vi "Utility Default Instrument Setup.vi"(0 "VISA resource name":refnum<visa-resource-name>, 11 "error in (no error)":errorcluster) -> (4 "VISA resource name out":refnum<visa-resource-name>, 15 "error out":errorcluster)   [LabVIEW 2016, in "Fluke 5XXX Series Multicalibrators.lvlib"]
doc: "This Utility VI sends a default command string to the instrument whenever a new VISA session is opened, or the instrument is reset. This VI is intended to be used as a subVI for the FL5XMCAL Initialize and FL5XMCAL Reset VI's. Altering this VI could cause these two VI's to operate incorrectly."
uses:
  Fluke 5XXX Series Multicalibrators.lvlib
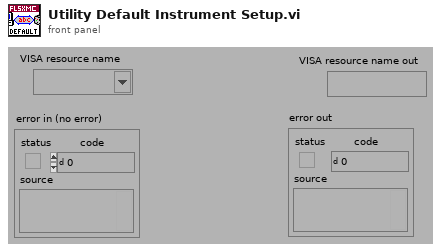
[diagram p1: front panel]
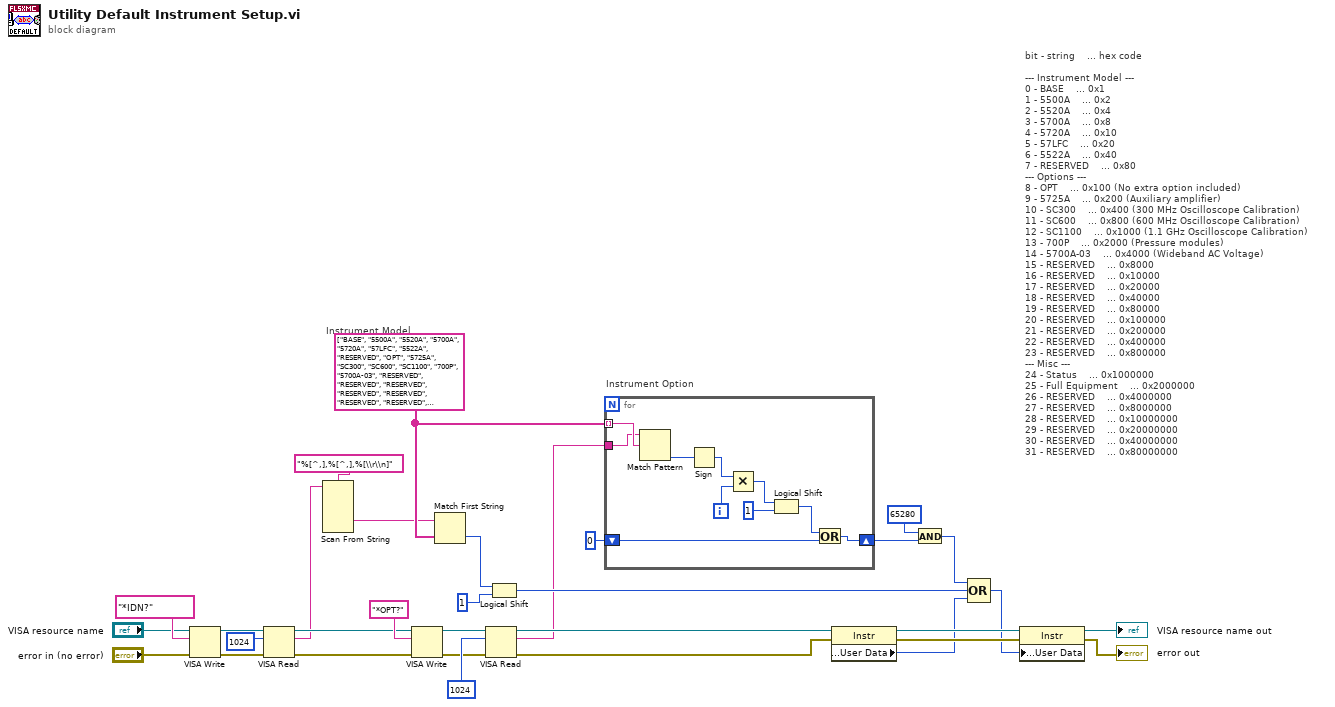
[diagram p0: block diagram]
diagram:
  w16 = string[] ["BASE", "5500A", "5520A", "5700A", "5720A", "57LFC", "5522A", "RESERVED", "OPT", "5725A", "SC300", "SC600", "SC1100", "700P", "5700A-03", "RESERVED", "RESERVED", "RESERVED", "RESERVED", "RESERVED", "RESERVED", "RESERVED", "RESERVED", "RESERVED", "Status", "Full Equipment", "RESERVED", "RESERVED", "RESERVED", "RESERVED", "RESERVED", "RESERVED", "525B"] ("Bits Array")
  # "bit - string    ... hex code\n\n--- Instrument Model ---\n0 - BASE    ... 0x1\n1 - 5500A    ... 0x2\n2 - 5520A    ... 0x4\n3 - 5700A    ... 0x8\n4 - 5720A    ... 0x10\n5 - 57LFC    ... 0x20\n6 - 5522A    ... 0x40\n7 - RESERVED    ... 0x80\n--- Options ---\n8 - OPT    ... 0x100 (No extra option included)\n9 - 5725A    ... 0x200 (Auxiliary amplifier)\n10 - SC300    ... 0x400 (300 MHz Oscilloscope Calibration)\n11 - SC600    ... 0x800 (600 MHz Oscilloscope Calibration)\n12 - SC1100    ... 0x1000 (1.1 GHz Oscilloscope Calibration)\n13 - 700P    ... 0x2000 (Pressure modules)\n14 - 5700A-03    ... 0x4000 (Wideband AC Voltage)\n15 - RESERVED    ... 0x8000\n16 - RESERVED    ... 0x10000\n17 - RESERVED    ... 0x20000\n18 - RESERVED    ... 0x40000\n19 - RESERVED    ... 0x80000\n20 - RESERVED    ... 0x100000\n21 - RESERVED    ... 0x200000\n22 - RESERVED    ... 0x400000\n23 - RESERVED    ... 0x800000\n--- Misc ---\n24 - Status    ... 0x1000000\n25 - Full Equipment    ... 0x2000000\n26 - RESERVED    ... 0x4000000\n27 - RESERVED    ... 0x8000000\n28 - RESERVED    ... 0x10000000\n29 - RESERVED    ... 0x20000000\n30 - RESERVED    ... 0x40000000\n31 - RESERVED    ... 0x80000000"
  # "Instrument Option"
  # "Instrument Model"
  n1 = VISA Write(VISA resource name="VISA resource name", write buffer="*IDN?" ("write buffer (\"\")"), error in (no error)="error in (no error)") -> (VISA resource name out=w31:refnum<visa-resource-name>, error out=w30:errorcluster)  [unwired: 1 out]
  n2 = VISA Read(VISA resource name=w31, byte count=u32 1024 ("byte count (0)"), error in (no error)=w30) -> (VISA resource name out=w23:refnum<visa-resource-name>, read buffer=w8:string, error out=w24:errorcluster)  [unwired: 1 out]
  n3 = Scan From String(format string="%[^,],%[^,],%[\\r\\n]" ("Format String"), input string=w8) -> (output 2=w6:string)  [unwired: 7 in, 3 out]
  n4 = VISA Write(VISA resource name=w23, write buffer="*OPT?" ("write buffer (\"\")"), error in (no error)=w24) -> (VISA resource name out=w26:refnum<visa-resource-name>, error out=w27:errorcluster)  [unwired: 1 out]
  n5 = Match First String(2:w16, 3:w6) -> (0:w7:i32)  [unwired: 1 out]
  n6 = VISA Read(VISA resource name=w26, byte count=u32 1024 ("byte count (0)"), error in (no error)=w27) -> (VISA resource name out=w11:refnum<visa-resource-name>, read buffer=w2:string, error out=w10:errorcluster)  [unwired: 1 out]
  n7 = Logical Shift(y=w7, x=u32 1 ("y")) -> (x << y=w3:u32)
  n8 = for {
    tunnel: w16 -> [w42] mode=indexing
    shift-right: [w35] -> w15
    shift-left: u32 0 -> [w36]
    tunnel: w2 -> [w34]
    i -> [w33]
    n9 = Match Pattern(string=w34, regular expression=w42) -> (offset past match=w38:i32)  [unwired: 1 in, 3 out]
    n10 = Sign(1:w38) -> (0:w40:i32)
    n11 = Multiply(x=w40, y=w33) -> (x*y=w39:i32)
    n12 = Logical Shift(y=w39, x=u32 1 ("y")) -> (x << y=w37:u32)
    n13 = Or(x=w37, y=w36) -> (x .or. y?=w35:u32)
  }
  n14 = property class="Instr"(reference=w11, error in=w10) -> (reference out=w13:refnum<visa-resource-name>, error out=w12:errorcluster, "General Settings:User Data"=w4:u32)
  n15 = And(x=u32 65280, y=w15) -> (x .and. y?=w9:u32)
  n16 = Compound Arithmetic op=OR(w9, w3, w4) -> (w1:u32)
  n17 = property class="Instr"(reference=w13, error in=w12, "General Settings:User Data"=w1) -> (reference out=→"VISA resource name out":refnum<visa-resource-name>, error out=→"error out":errorcluster)
